vi "read encoder test.vi"() -> ()   [LabVIEW 2019]
uses:
  <vilib>/WPC Systems Ltd/GECO Driver/Lib/GECOBase/GECO_Driver Class/GECO_SlotName.ctl
  <vilib>/WPC Systems Ltd/GECO Driver/Lib/GECOMotion/GECOMotion/_typedefine/Axis Select.ctl
  <vilib>/Platform/TimedLoop/XDataNode/timing_clust.ctl
  <vilib>/Platform/TimedLoop/XDataNode/nitl_modes.ctl
  <vilib>/Platform/TimedLoop/XDataNode/wakeup.ctl
  <vilib>/WPC Systems Ltd/GECO Driver/GECODriver/GECO_Initialize_RT/Initialize VIs/Initialize_GECOUnoRT_4HX.vi
  <vilib>/WPC Systems Ltd/GECO Driver/Lib/GECOMotion/GECOMotion/GECO Motion.lvclass
  <vilib>/platform/TimedLoop/XDataNode/XDataNode.xnode
  <vilib>/WPC Systems Ltd/GECO Driver/Lib/GECOBase/GECO_Driver Class/GECO_Driver.lvclass
  <vilib>/Platform/TimedLoop/XDataNode/XDNodeRunTimeDep.lvlib
panel:
  out "Period":u32
  out "Axis 3":T1
  out "Axis 2":T1
  out "Axis 1":T1
  in  "stop":bool
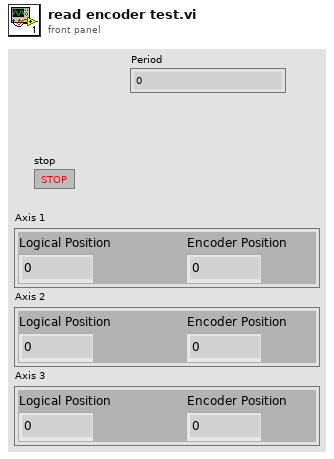
[diagram p1: front panel]
types:
  T1 = cluster{"Encoder Position":i32, "Logical Position":i32}
  T2 = typedef "GECO Motion.lvclass/Axis Select.ctl" = enum16{"Axis 1", "Axis 2", "Axis 3", "Axis 4"}
  T3 = typedef "GECO_Driver.lvclass/GECO_SlotName.ctl" = enum16{"C1", "C2", "C3", "C4"}
  T4 = typedef "XDNodeRunTimeDep.lvlib/timing_clust.ctl" = cluster{"Expected End [f-1]":u64, "Actual End [f-1]":u64, "Finished Late? [f-1]":bool, "Expected End [i-1]":u64, "Actual End [i-1]":u64, "Finished Late? [i-1]":bool, "Expected Start [i]":u64, "Actual Start [i]":u64, "Expected Start [f]":u64, "Actual Start [f]":u64, "Source Name":string, "Structure Name":string, "Period":i64, "Deadline":i64, "Offset":i64, "Start":i64, "Priority":i32, "Timeout":i32, "Mode":T5, "Wakeup Reason":T6, "Error":errorcluster, "Source Type":string, "Secondary Source Type":string, "Global End Time":u64, "Global Start Time":u64, "Frame Duration":u64, "Iteration Duration":u64, "Assigned CPU":i32, "I/O Scan Engine Mode":u32}
  T5 = typedef "XDNodeRunTimeDep.lvlib/nitl_modes.ctl" = enum32{"No Change", "Process missed periods, maintain original phase", "Discard missed periods, maintain original phase", "Process missed periods, ignore original phase", "Discard missed periods, ignore original phase"}
  T6 = typedef "XDNodeRunTimeDep.lvlib/wakeup.ctl" = enum32{"Normal", "Aborted", "Asynchronous wakeup", "Timing source error", "Timed loop error", "Timeout"}
  T7 = cluster{"Logical Position":i32, "Encoder Position":i32}
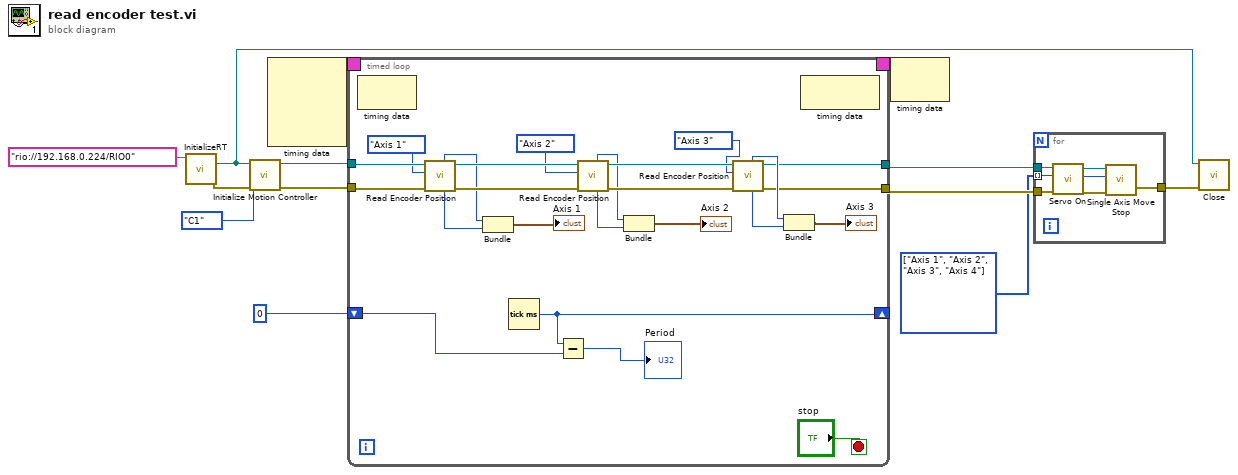
[diagram p0: block diagram]
diagram:
  w4 = T2[] [enum."Axis 1", enum."Axis 2", enum."Axis 3", enum."Axis 4"] items=["Axis 1", "Axis 2", "Axis 3", "Axis 4"]
  n1 = call-poly <vilib>:"InitializeRT.vi"("resource name"=tag "rio://192.168.0.224/RIO0") -> ("error out"=w12:errorcluster, "GECO_Driver out"=w2:refnum<class "GECO_Driver.lvclass">)  [unwired: 9 in]
  n2 = call <vilib>:"Initialize Motion Controller.vi"("error in (no error)"=w12, "Slot"=GECO_SlotName."C1", "GECO_Driver in"=w2) -> ("error out"=w7:errorcluster, "Motion reference out"=w8:refnum<class "GECO Motion.lvclass">)  [unwired: 7 in]
  n3 = node-c288() -> (w10:T4)  [unwired: 4 in]
  n4 = timed-loop {
    timing: w10 -> [_]
    timing-out: [_] -> w9
    tunnel: w8 -> [w31]
    tunnel: w7 -> [w32]
    tunnel: [w21] -> w6
    tunnel: [w20] -> w5
    shift-right: [w14] -> _
    shift-left: u32 0 ("millisecond timer value") -> [w15]
    stop <- "stop" stop-if-true
    n5 = node-c288() -> ()  [unwired: 1 in, 1 out]
    n6 = call <vilib>:"Read Encoder Position.vi"("error in (no error)"=w32, "Axis Select"=Axis_Select."Axis 1", "GECO Motion in"=w31) -> ("error out"=w35:errorcluster, "GECO Motion out"=w36:refnum<class "GECO Motion.lvclass">, "Encoder Position"=w29:i32, "Logical Position"=w30:i32)  [unwired: 4 in, 1 out]
    n7 = Bundle("Logical Position"=w30, "Encoder Position"=w29) -> (→"Axis 1":T7)  [unwired: 1 in]
    n8 = Tick Count (ms)() -> (millisecond timer value=w14:u32)
    n9 = Subtract(x=w14, y=w15) -> (x-y=→"Period":u32)
    n10 = call <vilib>:"Read Encoder Position.vi"("error in (no error)"=w35, "Axis Select"=Axis_Select."Axis 2", "GECO Motion in"=w36) -> ("error out"=w33:errorcluster, "GECO Motion out"=w34:refnum<class "GECO Motion.lvclass">, "Encoder Position"=w26:i32, "Logical Position"=w27:i32)  [unwired: 4 in, 1 out]
    n11 = Bundle("Logical Position"=w27, "Encoder Position"=w26) -> (→"Axis 2":T7)  [unwired: 1 in]
    n12 = call <vilib>:"Read Encoder Position.vi"("error in (no error)"=w33, "Axis Select"=Axis_Select."Axis 3", "GECO Motion in"=w34) -> ("error out"=w21:errorcluster, "GECO Motion out"=w20:refnum<class "GECO Motion.lvclass">, "Encoder Position"=w23:i32, "Logical Position"=w24:i32)  [unwired: 4 in, 1 out]
    n13 = Bundle("Logical Position"=w24, "Encoder Position"=w23) -> (→"Axis 3":T7)  [unwired: 1 in]
    n14 = node-c288() -> ()  [unwired: 1 in, 1 out]
  }
  n15 = node-c288(w9) -> ()  [unwired: 1 out]
  n16 = for {
    tunnel: w6 -> [w44]
    tunnel: w4 -> [w43] mode=indexing
    tunnel: w5 -> [w42]
    tunnel: [w40] -> w3
    n17 = call <vilib>:"Servo On.vi"("error in (no error)"=w44, "Axis Select"=w43, "GECO Motion in"=w42) -> ("error out"=w45:errorcluster, "Axis Select out"=w41:T2, "GECO Motion out"=w46:refnum<class "GECO Motion.lvclass">)  [unwired: 6 in]
    n18 = call <vilib>:"Single Axis Move Stop.vi"("error in (no error)"=w45, "Axis Select"=w41, "GECO Motion in"=w46) -> ("error out"=w40:errorcluster)  [unwired: 6 in, 2 out]
  }
  n19 = call <vilib>:"Close.vi"("error in (no error)"=w3, "GECO_Driver in"=w2) -> ()  [unwired: 9 in, 1 out]
